vi "AIT 1553 - Parse BM Sysdef Tree Messages.vi"(8 "error in":errorcluster, 9 "BM_Messages In":T2[](array[typedef]), 10 "Section Ptr":T1 format="%.0x") -> (0 "error out":errorcluster, 1 "BM_Messages Out":T2[](array[typedef]))   [LabVIEW 2013]
uses:
  <vilib>/NI Veristand/Custom Device API/Custom Device Item Ref.ctl
  Controls/1553_BM_Message.ctl
  Controls/664 -Param.ctl
  Controls and Global/Global.vi
  <vilib>/NI Veristand/Custom Device Tools/Custom Device Utility Library/NI VeriStand - Search for Item by Name.vi
  <vilib>/NI Veristand/Custom Device API/Get Item Property (I32).vi
  <vilib>/NI Veristand/Custom Device API/Get Item Property (Double).vi
  <vilib>/NI Veristand/Custom Device API/Get Item Property (Boolean).vi
  <vilib>/NI Veristand/Custom Device API/Custom Device API.lvlib
  AIT 664 Custom Device.lvlib
  <vilib>/NI Veristand/Custom Device Tools/Custom Device Utility Library/Custom Device Utility Library.lvlib
panel:
  out "Found":bool[](array[boolean])
  out "Property Names":string[][][](array[string])
  out "Channel Refs":T1[][](array[typedef]) format="%.0x"
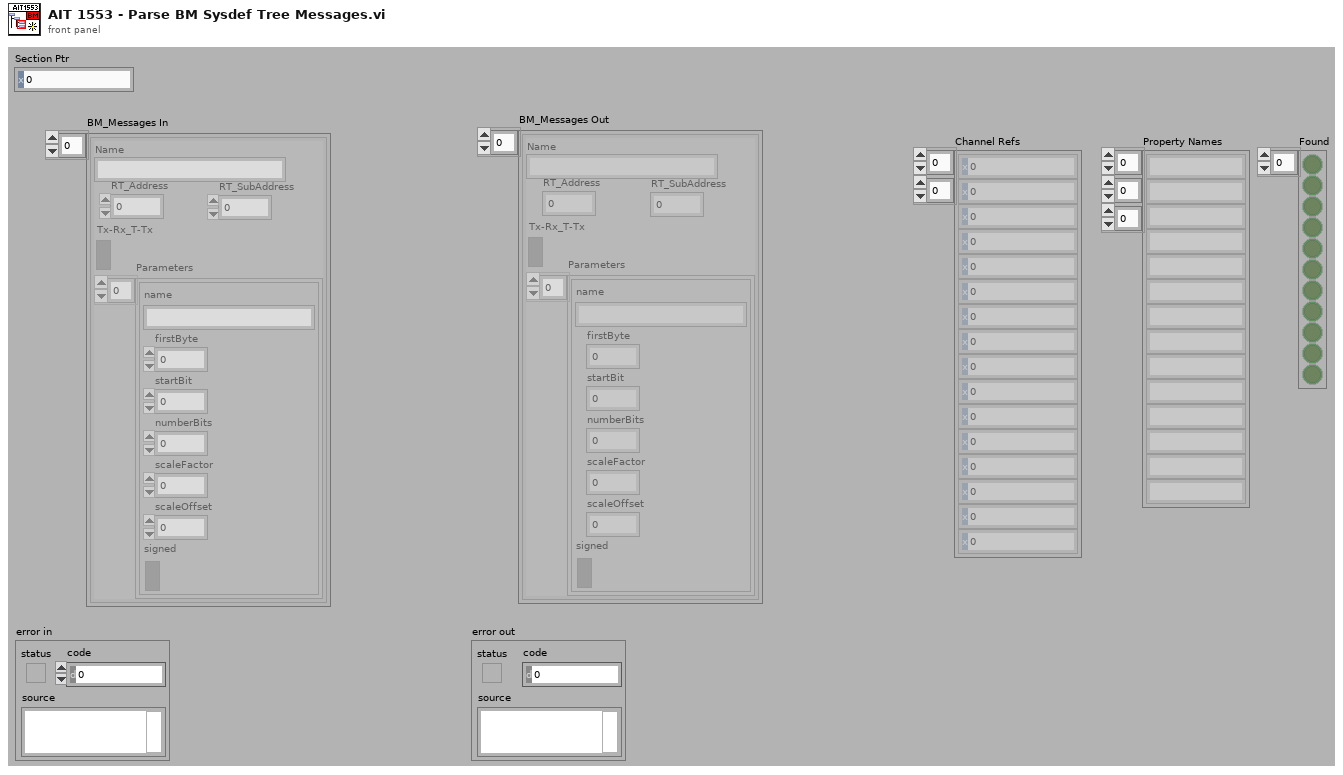
[diagram p1: front panel]
types:
  T1 = typedef "Custom Device API.lvlib/Custom Device Item Ref.ctl" = u64
  T2 = typedef "AIT 664 Custom Device.lvlib/1553_BM_Message.ctl" = cluster{"RT_Address":u8, "RT_SubAddress":u8, "Tx-Rx_T-Tx":bool, "Parameters":T3[], "Name":string}
  T3 = typedef "AIT 664 Custom Device.lvlib/664 -Param.ctl" = cluster{"name":string, "firstByte":i32, "startBit":i32, "numberBits":i32, "scaleFactor":dbl, "scaleOffset":dbl, "signed":bool}
  T4 = enum32{"Invalid", "Standard", "Closed", "Hidden", "Minimized", "Maximized"}
  T5 = typedef "Custom Device API.lvlib/Custom Device Item Info.ctl" = cluster{"Name":string, "Is Channel":bool, "GUID":string, "Is Waveform":bool}
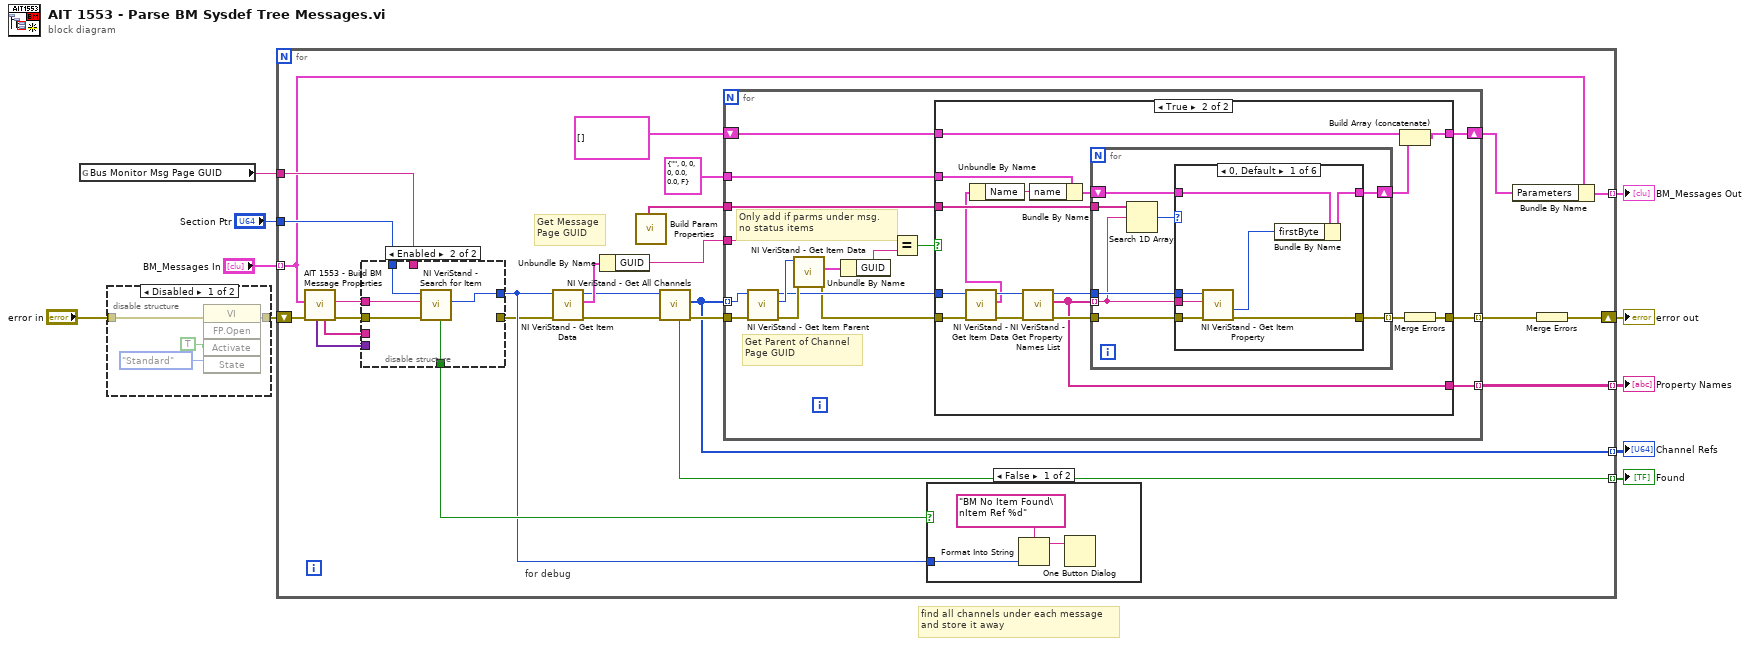
[diagram p0: block diagram]
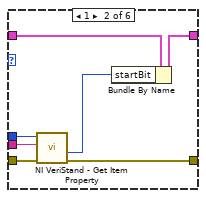
[diagram p5: hidden frame]
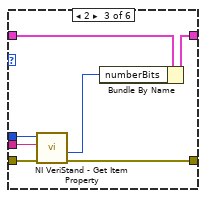
[diagram p6: hidden frame]
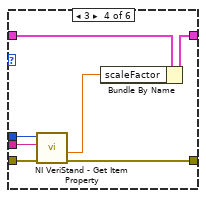
[diagram p7: hidden frame]
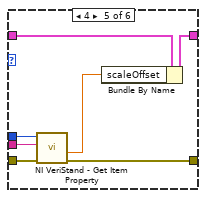
[diagram p8: hidden frame]
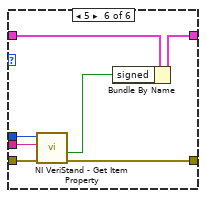
[diagram p9: hidden frame]
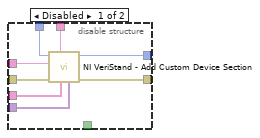
[diagram p10: hidden frame]
diagram:
  # "find all channels under each message\nand store it away"
  n1 = global read "Global.vi" "Bus Monitor Msg Page GUID"() -> (w8:string)
  n2 = disable-structure shown="Disabled" {
    disable-tunnel: "error in" -> [w12 w15]
    disable-tunnel: [w11 w15] -> w4
    frame Disabled {
      n3 = invoke class="VI" method="FP.Open"(error in=w12, "Activate"=TRUE ("Activate?"), "State"=T4."Standard") -> (error out=w11:errorcluster)  [unwired: 2 in, 4 out]
    }
    frame Enabled {
    }
  }
  n4 = for {
    shift-right: [w31] -> w10
    shift-left: w4 -> [w37]
    tunnel: "Section Ptr" -> [w35]
    tunnel: "BM_Messages In" -> [w24] mode=indexing
    tunnel: w8 -> [w36]
    tunnel: [w30] -> w6 mode=indexing
    tunnel: [w28] -> w3 mode=indexing
    tunnel: [w27] -> w2 mode=indexing
    tunnel: [w26] -> w1 mode=indexing
    # "Get Message\nPage GUID"
    # "for debug"
    n5 = call "AIT 1553 - Build BM Message Properties.vi"("error in (no error)"=w37, "BM_Message"=w24) -> ("error out"=w39:errorcluster, "name"=w38:string, "Prop Names"=w40:string[], "Prop Values"=w41:variant[])  [unwired: 5 in, 1 out]
    n6 = disable-structure shown="Enabled" {
      disable-tunnel: w41 -> [w137 _]
      disable-tunnel: w40 -> [w136 _]
      disable-tunnel: w39 -> [w135 w141]
      disable-tunnel: w38 -> [w134 w142]
      disable-tunnel: w36 -> [w133 _]
      disable-tunnel: w35 -> [w132 w140]
      disable-tunnel: [w131 _] -> w21
      disable-tunnel: [w130 w139] -> w22
      disable-tunnel: [_ w138] -> w29
      frame Disabled {
        n7 = call <vilib>:"NI VeriStand - Add Custom Device Section.vi"("Property Values"=w137, "Property names"=w136, "GUID (Default Section)"=w133, "error in (no error)"=w135, "Section Name"=w134, "Parent Ref in"=w132) -> ("error out"=w131:errorcluster, "Section Ptr"=w130:T1)  [unwired: 2 in, 2 out]
      }
      frame Enabled {
        n8 = call-poly <vilib>:"NI VeriStand - Search for Item.vi"("error in"=w141, "Item Name"=w142, "Section Ref in"=w140) -> ("Item Ref"=w139:T1, "Found"=w138:bool)  [unwired: 5 in, 2 out]
      }
    }
    n9 = call <vilib>:"NI VeriStand - Get Item Data.vi"("error in (no error)"=w21, "Item Ref in"=w22) -> ("error out"=w20:errorcluster, "Item Info"=w23:T5, "Item Ref out"=w19:T1)  [unwired: 6 in, 1 out]
    n10 = Unbundle By Name(w23) -> ("GUID"=w18:string)
    n11 = call "Build Param Properties.vi"() -> ("Prop Names"=w33:string[])  [unwired: 11 in, 8 out]
    n12 = call <vilib>:"NI VeriStand - Get All Channels.vi"("error in"=w20, "Section Ref in"=w19) -> ("error out"=w34:errorcluster, "Channel Refs"=w27:T1[], "Found"=w28:bool)  [unwired: 6 in, 1 out]
    n13 = for {
      tunnel: w34 -> [w52]
      tunnel: w27 -> [w51] mode=indexing
      tunnel: w33 -> [w60]
      tunnel: [w59] -> w32 mode=indexing
      tunnel: [w57] -> w26 mode=indexing
      tunnel: T3 {"name"="", "firstByte"=0, "startBit"=0, "numberBits"=0, "scaleFactor"=0.0, "scaleOffset"=0.0, "signed"=FALSE} ("1553 Parameter") -> [w58]
      tunnel: w18 -> [w48]
      shift-right: [w45] -> w16
      shift-left: T3[] [] -> [w47]
      # "Only add if parms under msg.\nno status items"
      # "Get Parent of Channel\nPage GUID"
      n14 = call <vilib>:"NI VeriStand - Get Item Parent.vi"("error in (no error)"=w52, "Item Ref in"=w51) -> ("error out"=w56:errorcluster, "Parent Ref"=w55:T1, "Item Ref out"=w50:T1)  [unwired: 6 in, 1 out]
      n15 = call <vilib>:"NI VeriStand - Get Item Data.vi"("error in (no error)"=w56, "Item Ref in"=w55) -> ("error out"=w49:errorcluster, "Item Info"=w54:T5)  [unwired: 6 in, 2 out]
      n16 = Unbundle By Name(w54) -> ("GUID"=w53:string)
      n17 = Equal?(x=w48, y=w53) -> (x = y?=w46:bool)
      n18 = case shown="True" w46 {
        tunnel: w60 -> [_ w78]
        tunnel: [w61 w75] -> w59
        tunnel: w58 -> [_ w72]
        tunnel: [_ w68] -> w57
        tunnel: w50 -> [_ w67]
        tunnel: w49 -> [w61 w66]
        tunnel: w47 -> [w62 w65]
        tunnel: [w62 w63] -> w45
        frame False {
        }
        frame True {
          n19 = call <vilib>:"NI VeriStand - Get Item Data.vi"("error in (no error)"=w66, "Item Ref in"=w67) -> ("error out"=w74:errorcluster, "Item Info"=w69:T5, "Item Ref out"=w73:T1)  [unwired: 6 in, 1 out]
          n20 = Unbundle By Name(w69) -> ("Name"=w70:string)
          n21 = call <vilib>:"NI VeriStand - Get Property Names List.vi"("error in (no error)"=w74, "Item Ref in"=w73) -> ("error out"=w79:errorcluster, "Property Names"=w68:string[], "Item Ref out"=w77:T1)  [unwired: 7 in]
          n22 = Bundle By Name(cluster=w72, "name"=w70) -> (w71:T3)
          n23 = for {
            tunnel: w79 -> [w84]
            tunnel: w68 -> [w82] mode=indexing
            tunnel: w78 -> [w87]
            shift-right: [w81] -> w64
            shift-left: w71 -> [w85]
            tunnel: w77 -> [w83]
            tunnel: [w80] -> w76 mode=indexing
            n24 = Search 1D Array(1D array=w87, element=w82) -> (index of element=w86:i32)  [unwired: 1 in]
            n25 = case shown="0, Default" w86 {
              tunnel: w85 -> [w94 w101 w108 w115 w122 w129]
              tunnel: w84 -> [w93 w100 w107 w114 w121 w128]
              tunnel: w83 -> [w92 w99 w106 w113 w120 w127]
              tunnel: w82 -> [w91 w98 w105 w112 w119 w126]
              tunnel: [w89 w96 w103 w110 w117 w124] -> w81
              tunnel: [w88 w95 w102 w109 w116 w123] -> w80
              frame 0, Default {
                n26 = call-poly <vilib>:"NI VeriStand - Get Item Property.vi"("error in (no error)"=w93, "Property Name"=w91, "Item Ref in"=w92) -> ("error out"=w88:errorcluster, "Value"=w90:i32)  [unwired: 5 in, 2 out]
                n27 = Bundle By Name(cluster=w94, "firstByte"=w90) -> (w89:T3)
              }
              frame 1 {
                n28 = call-poly <vilib>:"NI VeriStand - Get Item Property.vi"("error in (no error)"=w100, "Property Name"=w98, "Item Ref in"=w99) -> ("error out"=w95:errorcluster, "Value"=w97:i32)  [unwired: 5 in, 2 out]
                n29 = Bundle By Name(cluster=w101, "startBit"=w97) -> (w96:T3)
              }
              frame 2 {
                n30 = call-poly <vilib>:"NI VeriStand - Get Item Property.vi"("error in (no error)"=w107, "Property Name"=w105, "Item Ref in"=w106) -> ("error out"=w102:errorcluster, "Value"=w104:i32)  [unwired: 5 in, 2 out]
                n31 = Bundle By Name(cluster=w108, "numberBits"=w104) -> (w103:T3)
              }
              frame 3 {
                n32 = call-poly <vilib>:"NI VeriStand - Get Item Property.vi"("error in (no error)"=w114, "Property Name"=w112, "Item Ref in"=w113) -> ("error out"=w109:errorcluster, "Value"=w111:dbl)  [unwired: 5 in, 2 out]
                n33 = Bundle By Name(cluster=w115, "scaleFactor"=w111) -> (w110:T3)
              }
              frame 4 {
                n34 = call-poly <vilib>:"NI VeriStand - Get Item Property.vi"("error in (no error)"=w121, "Property Name"=w119, "Item Ref in"=w120) -> ("error out"=w116:errorcluster, "Value"=w118:dbl)  [unwired: 5 in, 2 out]
                n35 = Bundle By Name(cluster=w122, "scaleOffset"=w118) -> (w117:T3)
              }
              frame 5 {
                n36 = call-poly <vilib>:"NI VeriStand - Get Item Property.vi"("error in (no error)"=w128, "Property Name"=w126, "Item Ref in"=w127) -> ("error out"=w123:errorcluster, "Value"=w125:bool)  [unwired: 5 in, 2 out]
                n37 = Bundle By Name(cluster=w129, "signed"=w125) -> (w124:T3)
              }
            }
          }
          n38 = Build Array (concatenate)(w65, w64) -> (w63:T3[])
          n39 = Merge Errors(w76) -> (w75:errorcluster)
        }
      }
    }
    n40 = case shown="False" w29 {
      tunnel: w22 -> [w44 _]
      frame False {
        n41 = Format Into String(format string="BM No Item Found\nItem Ref %d" ("message"), w44) -> (resulting string=w43:string)  [unwired: 2 in, 1 out]
        n42 = One Button Dialog(message=w43) -> ()  [unwired: 1 in, 1 out]
      }
      frame True {
      }
    }
    n43 = Bundle By Name(cluster=w24, "Parameters"=w16) -> (w30:T2)
    n44 = Merge Errors(w32) -> (w31:errorcluster)
  }
  "error out" <- w10
  "BM_Messages Out" <- w6
  "Found" <- w3
  "Channel Refs" <- w2
  "Property Names" <- w1
